vi "closeLED.vi"(8 "error in (no error)":errorcluster, 11 "LED in":refnum<class "LED.lvclass">) -> (0 "error out":errorcluster)   [LabVIEW 2020, in "LED.lvclass"]
uses:
  LED.lvclass
  LED.lvclass/LED.ctl
  Sound/Sound.lvclass
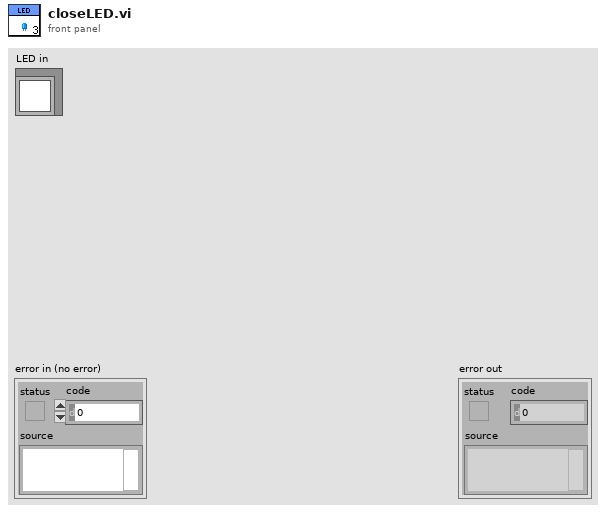
[diagram p1: front panel]
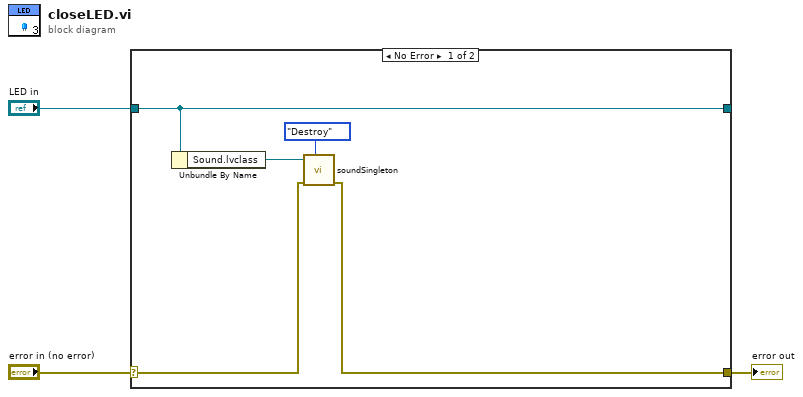
[diagram p0: block diagram]
diagram:
  n1 = case shown="No Error" "error in (no error)" {
    selector: "error in (no error)" -> [w5 w10]
    tunnel: [w4 w10] -> w2
    tunnel: [w8 w9] -> _
    tunnel: "LED in" -> [w8 w9]
    frame No Error {
      n2 = Unbundle By Name(w8) -> ("Sound.lvclass"=w7:refnum<class "Sound.lvclass">)
      n3 = call "soundSingleton.vi"("Option"=enum16{"Create", "Destroy"}."Destroy", "error in (no error)"=w5, "Sound in"=w7) -> ("error out"=w4:errorcluster)  [unwired: 7 in, 1 out]
    }
    frame Error {
    }
  }
  "error out" <- w2
